vi "Time and Date String.vi"(0 "Time (zero uses the current time)":dbl format="%.2f") -> (4 "date string":string, 8 "time string":string, 15 "date and time string":string)   [LabVIEW 2011]
panel:
  # "This vi returns the time and date strings. If the time control is zero (not wired) then the\nvi will use the current time instead"
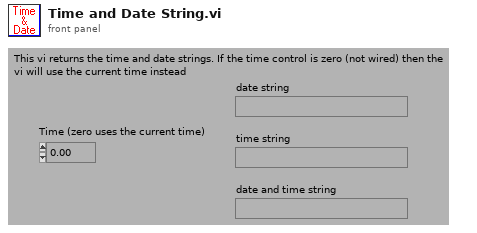
[diagram p1: front panel]
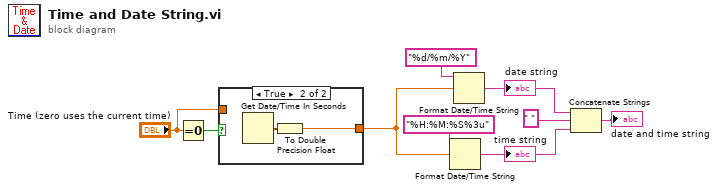
[diagram p0: block diagram]
diagram:
  n1 = Equal To 0?(x="Time (zero uses the current time)") -> (x = 0?=w6:bool)
  n2 = case shown="True" w6 {
    tunnel: [w10 w12] -> w8
    tunnel: "Time (zero uses the current time)" -> [w10 _]
    frame False {
    }
    frame True {
      n3 = Get Date/Time In Seconds() -> (seconds since 1Jan1904=w11:timestamp)
      n4 = To Double Precision Float(number=w11) -> (double precision float=w12:dbl)
    }
  }
  n5 = Format Date/Time String(time format string (%c)="%H:%M:%S%3u", seconds (now)=w8) -> (date/time string=w2:string)  [unwired: 1 in]
  "time string" <- w2
  n6 = Format Date/Time String(time format string (%c)="%d/%m/%Y", seconds (now)=w8) -> (date/time string=w3:string)  [unwired: 1 in]
  "date string" <- w3
  n7 = Concatenate Strings(w3, " ", w2) -> (→"date and time string":string)
